vi "Count Coins - Video.vi"() -> ()   [LabVIEW 2022 SP3]
uses:
  <vilib>/userdefined/High Color/IMAQdx.ctl
  <vilib>/vision/driver/NI_Vision_Acquisition_Software.lvlib
  Coin Analyser/Coin Analyser.lvclass
  <resource>/objmgr/imaqdx.rc
panel:
  out "Coins":i32
  out "Processed fps":dbl
  out "Coins":cluster{"x":i32, "y":i32, "diameter":i32}[](array[cluster])
  in  "stop":bool
  out "Image":T1(plugin-control)
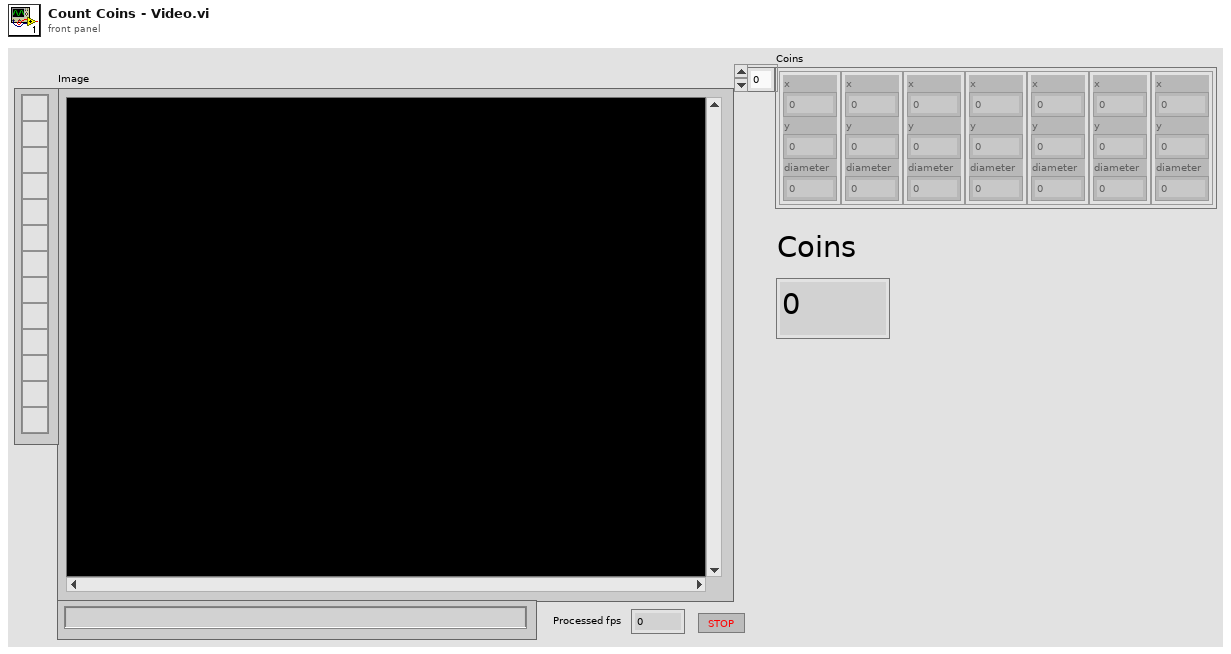
[diagram p1: front panel]
types:
  T1 = typedef "IMAQ Image.ctl" = refnum<image>
  T2 = typedef "IMAQdx.ctl" = refnum<k21>
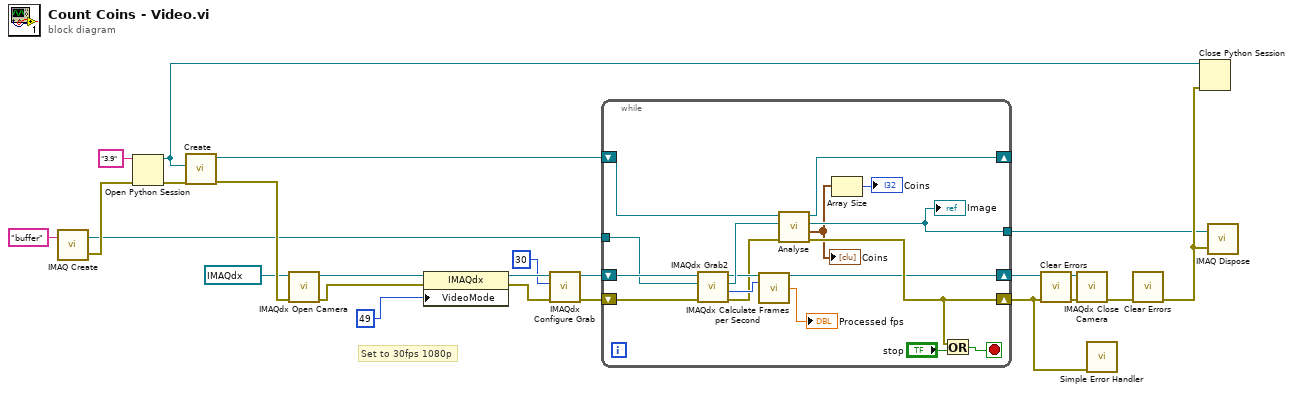
[diagram p0: block diagram]
diagram:
  # "Set to 30fps 1080p"
  n1 = call "IMAQ Create"("Image Name"="buffer") -> ("New Image"=w13:T1, "error out"=w21:errorcluster)  [unwired: 4 in]
  n2 = Open Python Session(python version="3.9" ("Python version"), 3:w21) -> (session out=w17:refnum<k35>, error out=w20:errorcluster)  [unwired: 1 in]
  n3 = call "Create.vi"("error in (no error)"=w20, "session"=w17) -> ("error out"=w19:errorcluster, "Coin Analyser out"=w18:refnum<class "Coin Analyser.lvclass">)  [unwired: 8 in]
  n4 = call <vilib>:"IMAQdx Open Camera.vi"("error in"=w19, "Session In"=T2 "cam0") -> ("error out"=w4:errorcluster, "Session Out"=w5:T2)  [unwired: 8 in]
  n5 = property class="IMAQdx"(reference=w5, error in=w4, "VideoMode"=u32 49) -> (reference out=w7:T2, error out=w6:errorcluster)
  n6 = call <vilib>:"IMAQdx Configure Grab.vi"("error in"=w6, "Number of Buffers"=u32 30, "Session In"=w7) -> ("error out"=w14:errorcluster, "Session Out"=w15:T2)  [unwired: 7 in]
  n7 = while {
    tunnel: w13 -> [w37]
    shift-right: [w30] -> w12
    shift-left: w15 -> [w39]
    shift-right: [w33] -> w10
    shift-left: w14 -> [w38]
    shift-right: [w32] -> _
    shift-left: w18 -> [w40]
    tunnel: [w27] -> w2
    stop <- w34 stop-if-true
    n8 = call <vilib>:"IMAQdx Grab2.vi"("error in"=w38, "Image In"=w37, "Session In"=w39) -> ("error out"=w26:errorcluster, "Buffer Number Out"=w29:u32, "Image Out"=w36:T1, "Session Out"=w31:T2)  [unwired: 5 in]
    n9 = call <vilib>:"IMAQdx Calculate Frames per Second.vi"("Session In"=w31, "Buffer Number"=w29) -> ("Session Out"=w30:T2, "Processed Frames per Second"=→"Processed fps":dbl)  [unwired: 7 in, 5 out]
    n10 = call "Analyse.vi"("error in (no error)"=w26, "Image in"=w36, "Coin Analyser in"=w40) -> ("error out"=w33:errorcluster, "Coins"=w25:cluster{"x":i32, "y":i32, "diameter":i32}[], "Image Out"=w27:T1, "Coin Analyser out"=w32:refnum<class "Coin Analyser.lvclass">)  [unwired: 5 in]
    "Image" <- w27
    "Coins" <- w25
    n11 = Array Size(array=w25) -> (size(s)=→"Coins":i32)
    n12 = Or(x=w33, y="stop") -> (x .or. y?=w34:bool)
  }
  n13 = call <vilib>:"Clear Errors.vi"("error in (no error)"=w10) -> ("error out"=w9:errorcluster)  [unwired: 5 in, 1 out]
  n14 = call <vilib>:"IMAQdx Close Camera.vi"("error in"=w9, "Session In"=w12) -> ("error out"=w11:errorcluster)  [unwired: 9 in]
  n15 = call <vilib>:"Simple Error Handler.vi"("error in (no error)"=w10) -> ()  [unwired: 4 in, 5 out]
  n16 = call <vilib>:"Clear Errors.vi"("error in (no error)"=w11) -> ("error out"=w3:errorcluster)  [unwired: 5 in, 1 out]
  n17 = Close Python Session(session in=w17, error in=w3) -> ()  [unwired: 1 out]
  n18 = call "IMAQ Dispose"("Image"=w2, "error in (no error)"=w3) -> ()  [unwired: 4 in, 1 out]
